vi "tdmsLiveCreation.vi"() -> ()   [LabVIEW 2026]
uses:
  <vilib>/Platform/TimedLoop/XDataNode/nitl_modes.ctl
  <vilib>/Platform/TimedLoop/XDataNode/timing_clust.ctl
  <vilib>/Platform/TimedLoop/XDataNode/wakeup.ctl
  <vilib>/platform/TimedLoop/XDataNode/XDataNode.xnode
  <vilib>/DAQmx/configure/task.llb/DAQmx Configure Logging (TDMS).vi
  <vilib>/DAQmx/create/channels.llb/DAQmx Create Channel (AI-Voltage-Basic).vi
  <vilib>/DAQmx/configure/timing.llb/DAQmx Timing (Sample Clock).vi
  <vilib>/Platform/TimedLoop/XDataNode/XDNodeRunTimeDep.lvlib
panel:
  out "10 second countdown":dbl
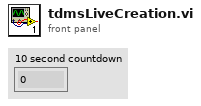
[diagram p1: front panel]
types:
  T1 = typedef "XDNodeRunTimeDep.lvlib/nitl_modes.ctl" = enum32{"No Change", "Process missed periods, maintain original phase", "Discard missed periods, maintain original phase", "Process missed periods, ignore original phase", "Discard missed periods, ignore original phase"}
  T2 = typedef "XDNodeRunTimeDep.lvlib/timing_clust.ctl" = cluster{"Expected End [f-1]":u64, "Actual End [f-1]":u64, "Finished Late? [f-1]":bool, "Expected End [i-1]":u64, "Actual End [i-1]":u64, "Finished Late? [i-1]":bool, "Expected Start [i]":u64, "Actual Start [i]":u64, "Expected Start [f]":u64, "Actual Start [f]":u64, "Source Name":string, "Structure Name":string, "Period":i64, "Deadline":i64, "Offset":i64, "Start":i64, "Priority":i32, "Timeout":i32, "Mode":T1, "Wakeup Reason":T3, "Error":errorcluster, "Source Type":string, "Secondary Source Type":string, "Global End Time":u64, "Global Start Time":u64, "Frame Duration":u64, "Iteration Duration":u64, "Assigned CPU":i32, "I/O Scan Engine Mode":u32}
  T3 = typedef "XDNodeRunTimeDep.lvlib/wakeup.ctl" = enum32{"Normal", "Aborted", "Asynchronous wakeup", "Timing source error", "Timed loop error", "Timeout"}
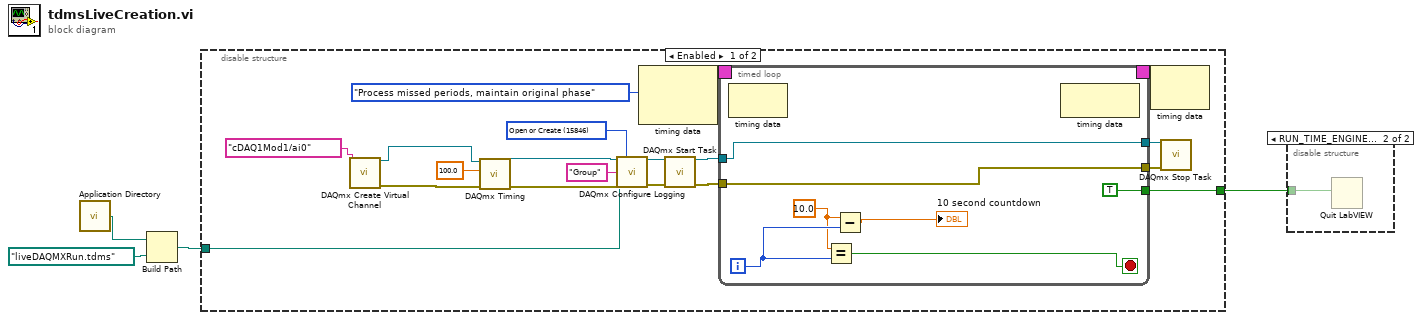
[diagram p0: block diagram]
diagram:
  n1 = call <vilib>:"Application Directory.vi"() -> ("Application Directory"=w3:path)
  n2 = Build Path(base path=w3, name or relative path=path "liveDAQMXRun.tdms") -> (appended path=w2:path)
  n3 = disable-structure shown="Enabled" {
    disable-tunnel: w2 -> [w9 _]
    disable-tunnel: [w6 _] -> w1
    frame Enabled {
      w20 = 15846 items=["Open"=10437, "Open or Create"=15846, "Create or Replace"=15847, "Create"=15848] ("operation")
      n4 = call-poly <vilib>:"DAQmx Create Virtual Channel.vi"("physical channels"=tag "cDAQ1Mod1/ai0") -> ("task out"=w8:refnum<k21>, "error out"=w7:errorcluster)  [unwired: 13 in]
      n5 = call-poly <vilib>:"DAQmx Timing.vi"("task/channels in"=w8, "rate"=100.0, "error in"=w7) -> ("task out"=w18:refnum<k21>, "error out"=w17:errorcluster)  [unwired: 11 in]
      n6 = call-poly <vilib>:"DAQmx Configure Logging.vi"("task/channels in"=w18, "operation"=w20, "file path"=w9, "group name"="Group", "error in"=w17) -> ("task out"=w16:refnum<k21>, "error out"=w15:errorcluster)  [unwired: 9 in]
      n7 = node-c288(nitl_modes."Process missed periods, maintain original phase" ("Mode")) -> (w23:T2)  [unwired: 1 in]
      n8 = call <vilib>:"DAQmx Start Task.vi"("task/channels in"=w16, "error in"=w15) -> ("task out"=w14:refnum<k21>, "error out"=w13:errorcluster)  [unwired: 12 in]
      n9 = timed-loop {
        tunnel: w14 -> [w29]
        tunnel: w13 -> [w28]
        timing: w23 -> [_]
        timing-out: [_] -> w22
        tunnel: [w29] -> w12
        tunnel: [w28] -> w11
        tunnel: [TRUE ("quit? (T)")] -> w6
        i -> [w26]
        stop <- w30 stop-if-true
        w24 = 10.0 ("x")
        n10 = node-c288() -> ()  [unwired: 1 in, 1 out]
        n11 = Equal?(x=w24, y=w26) -> (x = y?=w30:bool)
        n12 = Subtract(x=w24, y=w26) -> (x-y=→"10 second countdown":dbl)
        n13 = node-c288() -> ()  [unwired: 1 in, 1 out]
      }
      n14 = node-c288(w22) -> ()  [unwired: 1 out]
      n15 = call <vilib>:"DAQmx Stop Task.vi"("task/channels in"=w12, "error in"=w11) -> ()  [unwired: 12 in, 2 out]
    }
    frame Disabled {
    }
  }
  n16 = disable-structure shown="RUN_TIME_ENGINE==True" {
    disable-tunnel: w1 -> [_ w37]
    frame condition #0 (active) {
    }
    frame condition #1 {
      n17 = Quit LabVIEW(quit? (T)=w37) -> ()
    }
  }
